vi "Erase Program.vi"(4 "error in (no error)":errorcluster, 6 "Program # (1)":i32=1 min=0 max=100, 7 "VISA resource name":refnum<visa-resource-name>) -> (0 "error out":errorcluster, 3 "VISA resource name out":refnum<visa-resource-name>)   [LabVIEW 2019, in "Newport ESP301.lvlib"]
doc: "This command makes the program xx loaded in controller’s non-volatile memory unavailable to user. It does not delete the program from memory. Consequently, the program space does not become available to user immediately after deleting the program. It becomes available to user only after the entire stored program memory is purged by issuing this command with Program#=0.\n<B>Note:</B> Purging the stored program memory takes approximately 3 seconds for completion."
uses:
  Newport ESP301.lvlib
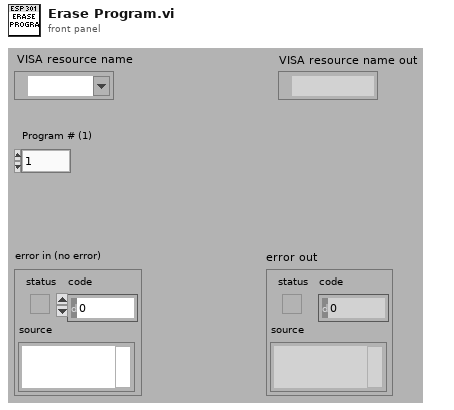
[diagram p1: front panel]
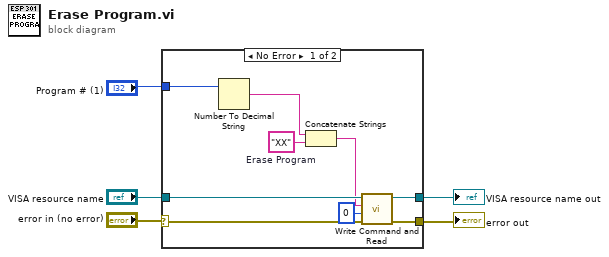
[diagram p0: block diagram]
diagram:
  n1 = case shown="No Error" "error in (no error)" {
    selector: "error in (no error)" -> [w11 w16]
    tunnel: [w13 w16] -> w5
    tunnel: "VISA resource name" -> [w14 w15]
    tunnel: [w12 w15] -> w4
    tunnel: "Program # (1)" -> [w7 _]
    frame No Error {
      w10 = "XX"  # Erase Program
      n2 = Number To Decimal String(number=w7) -> (decimal integer string=w9:string)  [unwired: 1 in]
      n3 = Concatenate Strings(w9, w10) -> (w8:string)
      n4 = call "Write Command and Read.vi"("error in (no error)"=w11, "Bytes to read (100)"=u32 0, "Command"=w8, "VISA resource name"=w14) -> ("error out"=w13:errorcluster, "VISA resource name out"=w12:refnum<visa-resource-name>)  [unwired: 3 in, 1 out]
    }
    frame Error {
    }
  }
  "error out" <- w5
  "VISA resource name out" <- w4
